vi "TEST - Get Frontmost VI.vi"(8 "error in (no error)":errorcluster) -> (0 "error out":errorcluster, 2 "pass":bool)   [LabVIEW 2009]
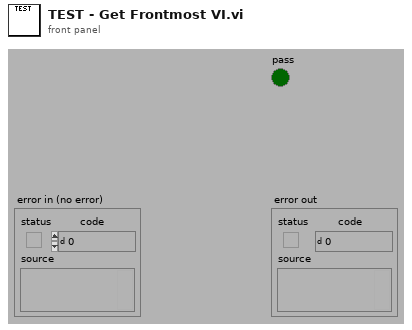
[diagram p1: front panel]
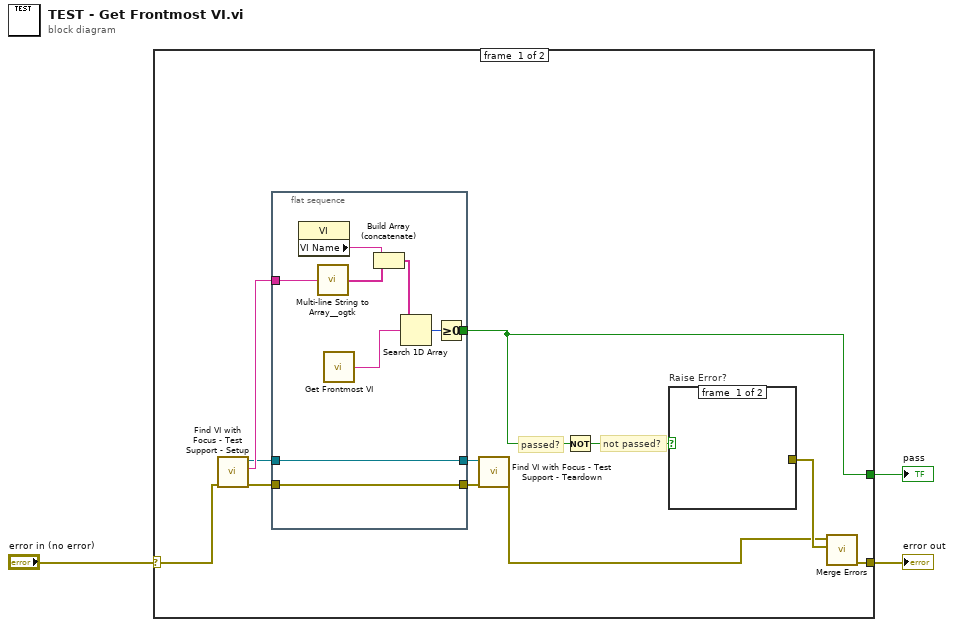
[diagram p0: block diagram]
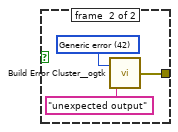
[diagram p2: hidden frame]
diagram:
  n1 = case shown="No Error" "error in (no error)" {
    selector: "error in (no error)" -> [w10 w27]
    tunnel: [w11 _] -> w3
    tunnel: [w14 w27] -> w1
    frame #0 {
      # "not passed?"
      # "passed?"
      n2 = call "Find VI with Focus - Test Support - Setup.vi"("error in (no error)"=w10) -> ("error out"=w4:errorcluster, "VI Name"=w8:string, "VI Renum"=w6:refnum<vi>)  [unwired: 8 in]
      n3 = flat-sequence {
        tunnel: [w22] -> w11
        tunnel: w8 -> [w17]
        tunnel: [w16] -> w7
        tunnel: w6 -> [w16]
        tunnel: [w15] -> w5
        tunnel: w4 -> [w15]
        frame #0 {
          n4 = property class="VI"() -> ("VI Name"=w21:string)  [unwired: 2 in, 2 out]
          n5 = call <userlib>:"Multi-line String to Array__ogtk.vi"("string"=w17) -> ("lines"=w20:string[])
          n6 = call "Get Frontmost VI.vi"() -> ("VI Name"=w18:string)
          n7 = Build Array (concatenate)(w21, w20) -> (w19:string[])
          n8 = Search 1D Array(1D array=w19, element=w18) -> (index of element=w23:i32)  [unwired: 1 in]
          n9 = Greater Or Equal To 0?(x=w23) -> (x >= 0?=w22:bool)
        }
      }
      n10 = call "Find VI with Focus - Test Support - Teardown.vi"("error in (no error)"=w5, "VI Renum"=w7) -> ("error out"=w9:errorcluster)  [unwired: 9 in]
      n11 = Not(x=w11) -> (.not. x?=w12:bool)
      n12 = case "Raise Error?" shown="True" w12 {
        tunnel: [_ w24] -> w13
        frame #0 {
        }
        frame #1 {
          w25 = 42 items=["No error", "Argument error", "Memory is full", "Out of zone", "End of file", "File already open", "Generic file I/O error", "File not found", "File permission error", "Disk is full", "Duplicate path", "Too many files open", "System feature not enabled", "Resource file not found", "Cannot add resource", "Resource not found", "Image not found", "Image memory error", "Pen does not exist", "Config type invalid", "Config token not found", "Config parse error", "Config memory error", "Bad external code format", "Bad external code offset", "External code not present", "Null window", "Destroy window error", "Null menu", "Print aborted", "Bad print record", "Print driver error", "Windows error during printing", "Memory error during printing", "Print dialog error", "Generic print error", "Invalid device refnum", "Device not found", "Device parameter error", "Device unit error", "Cannot open device", "Device call aborted", "Generic error", "Cancelled by user", "Object ID too low", "Object ID too high", "Object not in heap", "Unknown heap", "Unknown object (invalid DefProc)", "Unknown object (DefProc not in table)", "Message out of range", "Invalid (null) method", "Unknown message", "Manager call not supported", "Bad address", "Network operation in progress", "Network operation timed out", "Connection is busy", "Network attribute not supported", "Network error", "Address in use", "System out of memory", "Connection aborted", "Connection refused", "Not connected", "Already connected", "Connection closed", "Initialization error (interapplication manager)", "Bad occurrence", "Wait on unbound occurrence handler", "Occurrence queue overflow", "Datalog type conflict", "Unused", "Unrecognized type (interapplication manager)", "Memory corrupt", "Failed to make temporary DLL", "Old CIN version", "Drag socket not found", "Failed to load drop-object", "Failed to register OLE object", "Failed to release OLE object", "Format specifier type mismatch", "Unknown format specifier", "Too few format specifiers", "Too many format specifiers", "Scan failed", "Newer CIN version", "Error converting to variant", "Runtime menu error", "Password tampered", "Variant attribute not found", "Incompatible variant data type", "Event data is not available", "Event Store is not present", "Occurrence is not found", "Event Queue is not created", "Event info is not available", "Refnum passed is NULL", "Error retrieving Class GUID", "Error retrieving CoClass GUID", "Error retrieving TypeLib GUID.", "Bad built application magic bytes.", "Specific driver is different from the specific driver associated with the Logical Name.", "There is no session opened to the class driver.", "Max Error", "MAX - Error with config objects", "MAX - Error loading configuration", "MAX - Group not supported"]
          n13 = call <userlib>:"Build Error Cluster__ogtk.vi"("String to Prepend to source (\"\")"="unexpected output" ("String to Prepend to source (\"\")"), "code"=w25) -> ("error out"=w24:errorcluster)
        }
      }
      n14 = call <vilib>:"Merge Errors.vi"("error in 2 (no error)"=w13, "error in 1 (no error)"=w9) -> ("error out"=w14:errorcluster)  [unwired: 5 in]
    }
    frame #1 {
    }
  }
  "pass" <- w3
  "error out" <- w1
